vi "Util_WheelSpeedCalculations.vi"(11 "Sonar Distance":dbl) -> (3 "Wheel RPM":dbl)   [LabVIEW 2017, in "Shooter.lvlib"]
uses:
  Shooter.lvlib
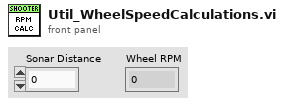
[diagram p1: front panel]
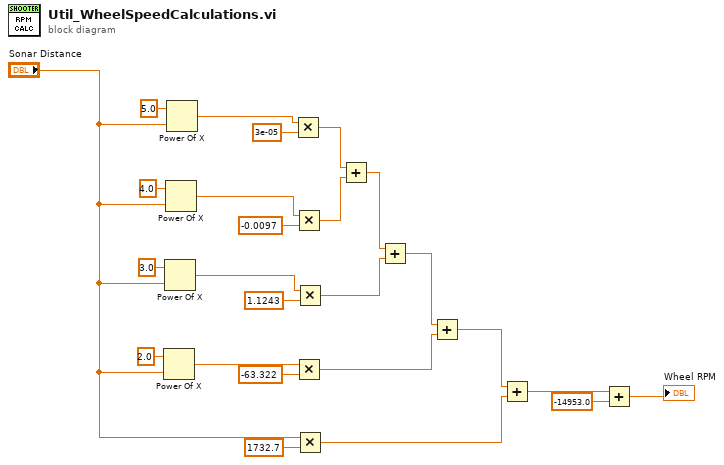
[diagram p0: block diagram]
diagram:
  n1 = Power Of X(1:"Sonar Distance", 2:2.0 ("y")) -> (0:w3:dbl)
  n2 = Power Of X(1:"Sonar Distance", 2:3.0 ("y")) -> (0:w20:dbl)
  n3 = Power Of X(1:"Sonar Distance", 2:4.0 ("y")) -> (0:w21:dbl)
  n4 = Power Of X(1:"Sonar Distance", 2:5.0 ("y")) -> (0:w22:dbl)
  n5 = Multiply(x=w22, y=3e-05) -> (x*y=w15:dbl)
  n6 = Multiply(x=w21, y=-0.0097) -> (x*y=w14:dbl)
  n7 = Multiply(x=w3, y=-63.322) -> (x*y=w10:dbl)
  n8 = Multiply(x=w20, y=1.1243) -> (x*y=w12:dbl)
  n9 = Multiply(x="Sonar Distance", y=1732.7) -> (x*y=w5:dbl)
  n10 = Add(x=w15, y=w14) -> (x+y=w13:dbl)
  n11 = Add(x=w13, y=w12) -> (x+y=w11:dbl)
  n12 = Add(x=w11, y=w10) -> (x+y=w7:dbl)
  n13 = Add(x=w7, y=w5) -> (x+y=w6:dbl)
  n14 = Add(x=w6, y=-14953.0) -> (x+y=→"Wheel RPM":dbl)
